vi "Project.Items.Add.vi"(8 "error in (no error)":errorcluster, 9 "Array":T1(array[cluster]), 10 "FPGA Target Name":string="FPGA Target", 11 "Path":path=path "C:/Users/Administrator/Desktop/Test Adding Memory to Project.lvproj") -> (0 "error out":errorcluster)   [LabVIEW 2015]
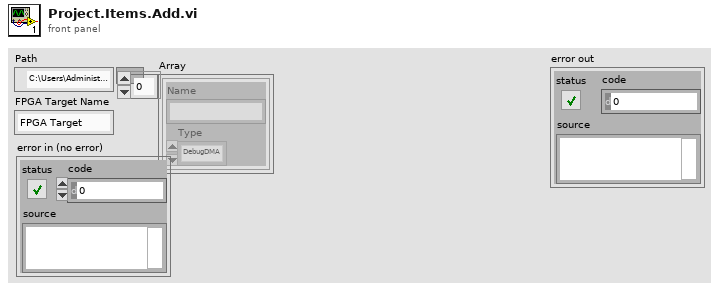
[diagram p1: front panel]
types:
  T1 = cluster{"Name":string, "Type":enum16{"DebugDMA", "Directional Memory", "Analog Replay Memory", "Pattern Generation Memory"}}[]
  T2 = enum16{"DebugDMA", "Directional Memory", "Analog Replay Memory", "Pattern Generation Memory"}
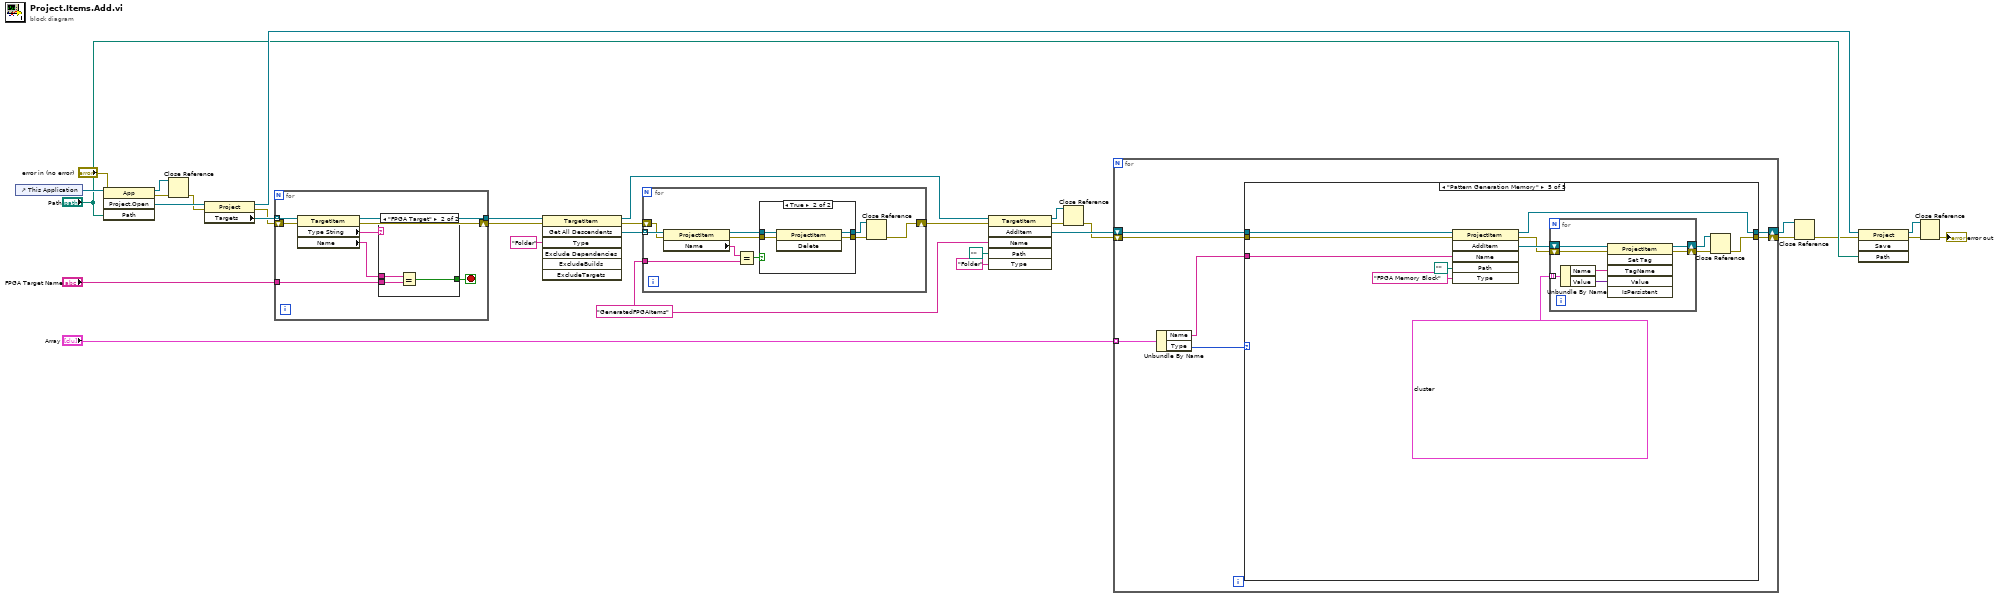
[diagram p0: block diagram]
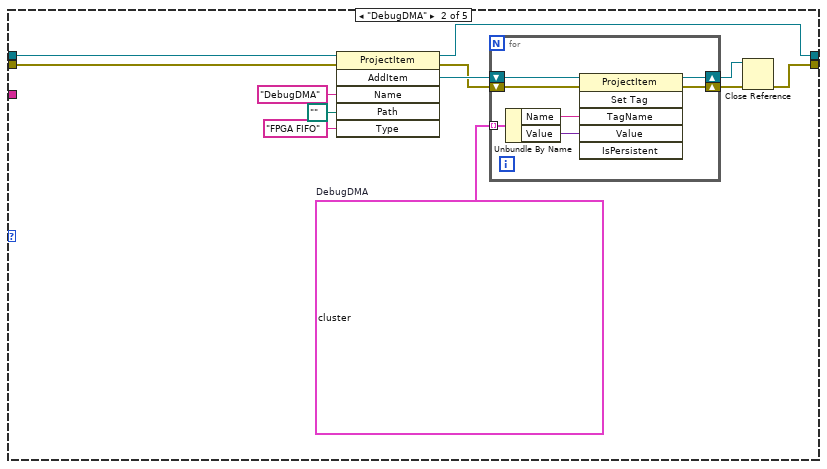
[diagram p3: hidden frame]
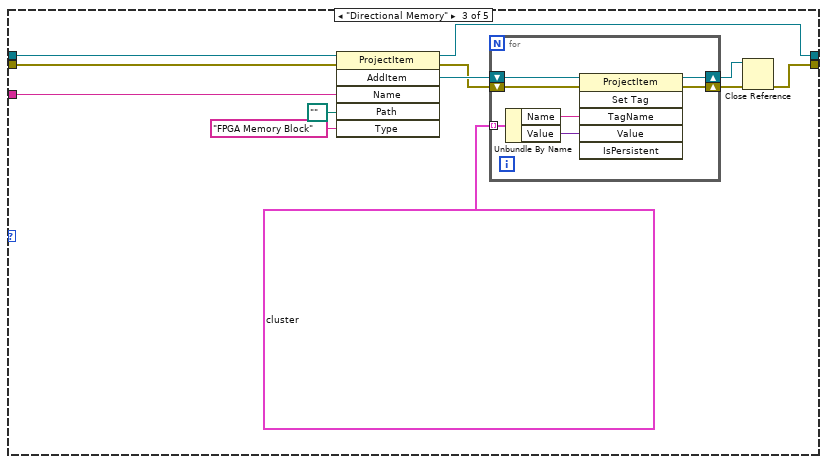
[diagram p4: hidden frame]
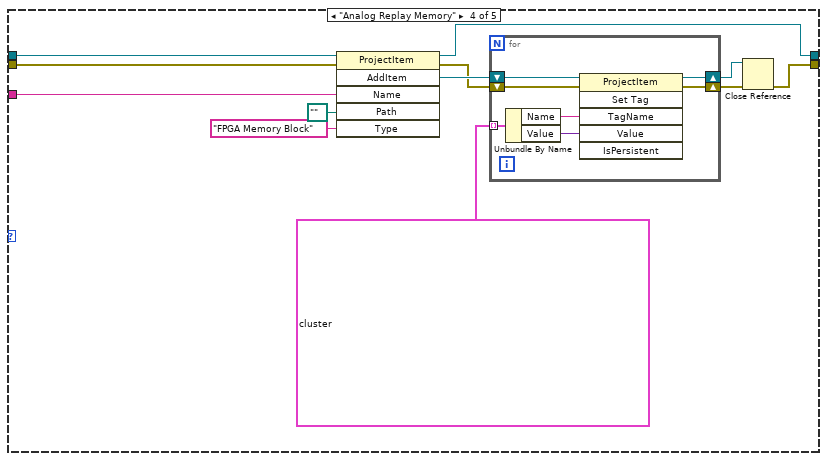
[diagram p5: hidden frame]
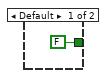
[diagram p6: hidden frame]
diagram:
  w12 = "GeneratedFPGAItems" ("Name")
  n1 = control-ref of="This Application"() -> (w32:refnum<vi>)
  n2 = invoke class="App" method="Project.Open"(reference=w32, error in="error in (no error)", "Path"="Path") -> (reference out=w19:refnum<vi>, error out=w21:errorcluster, "Project:Open"=w31:refnum<vi>)  [unwired: 1 in, 1 out]
  n3 = Close Reference(reference=w19, error in (no error)=w21) -> (error out=w20:errorcluster)
  n4 = property class="Project"(reference=w31, error in=w20) -> (reference out=w26:refnum<vi>, error out=w17:errorcluster, "Targets"=w18:refnum<vi>[])
  n5 = for {
    tunnel: w18 -> [w40] mode=indexing
    tunnel: "FPGA Target Name" -> [w39]
    shift-right: [w36] -> w16
    shift-left: w17 -> [w37]
    tunnel: [w35] -> w15
    stop <- w34 stop-if-true
    n6 = property class="TargetItem"(reference=w40, error in=w37) -> (reference out=w35:refnum<vi>, error out=w36:errorcluster, "Type String"=w33:string, "Name"=w38:string)
    n7 = case shown="\"FPGA Target\"" w33 {
      tunnel: w39 -> [_ w44]
      tunnel: w38 -> [_ w43]
      tunnel: [FALSE w42] -> w34
      frame Default {
      }
      frame "FPGA Target" {
        n8 = Equal?(x=w43, y=w44) -> (x = y?=w42:bool)
      }
    }
  }
  n9 = invoke class="TargetItem" method="Get All Descendents"(reference=w15, error in=w16, "Type"="Folder") -> (reference out=w13:refnum<vi>, error out=w22:errorcluster, "All Descendents"=w23:refnum<vi>[])  [unwired: 4 in, 4 out]
  n10 = for {
    tunnel: w23 -> [w54] mode=indexing
    shift-right: [w45] -> w28
    shift-left: w22 -> [w53]
    tunnel: w12 -> [w51]
    n11 = property class="ProjectItem"(reference=w54, error in=w53) -> (reference out=w50:refnum<vi>, error out=w49:errorcluster, "Name"=w52:string)
    n12 = Equal?(x=w52, y=w51) -> (x = y?=w48:bool)
    n13 = case shown="True" w48 {
      tunnel: w50 -> [w55 w60]
      tunnel: w49 -> [w56 w59]
      tunnel: [w56 w58] -> w46
      tunnel: [w55 w57] -> w47
      frame False {
      }
      frame True {
        n14 = invoke class="ProjectItem" method="Delete"(reference=w60, error in=w59) -> (reference out=w57:refnum<vi>, error out=w58:errorcluster)  [unwired: 1 in, 1 out]
      }
    }
    n15 = Close Reference(reference=w47, error in (no error)=w46) -> (error out=w45:errorcluster)
  }
  n16 = invoke class="TargetItem" method="AddItem"(reference=w13, error in=w28, "Name"=w12, "Path"=path "", "Type"="Folder") -> (reference out=w11:refnum<vi>, error out=w10:errorcluster, "AddItem"=w29:refnum<vi>)  [unwired: 1 in, 3 out]
  n17 = Close Reference(reference=w11, error in (no error)=w10) -> (error out=w9:errorcluster)
  n18 = for {
    shift-right: [w66] -> w5
    shift-left: w9 -> [w65]
    shift-right: [w64] -> w3
    shift-left: w29 -> [w67]
    tunnel: "Array" -> [w63] mode=indexing
    n19 = Unbundle By Name(w63) -> ("Name"=w61:string, "Type"=w62:T2)
    n20 = case shown="\"Pattern Generation Memory\"" w62 {
      tunnel: w67 -> [w68 w81 w100 w119 w138]
      tunnel: [w69 w70 w92 w111 w130] -> w66
      tunnel: w65 -> [w69 w75 w90 w108 w128]
      tunnel: [w68 w73 w95 w114 w133] -> w64
      tunnel: w61 -> [_ _ w89 w109 w127]
      frame Default {
      }
      frame "DebugDMA" {
        w77 = cluster{"Name":string, "Value":variant}[] [{"Name"="Actual Number of Elements", "Value"=variant(u32 1023)}, {"Name"="Arbitration for Read", "Value"=variant(u32 1)}, {"Name"="Arbitration for Write", "Value"=variant(u32 1)}, {"Name"="Control Logic", "Value"=variant(u32 0)}, {"Name"="Data Type", "Value"=variant(u32 11)}, {"Name"="Disable on Overflow/Underflow", "Value"=variant(bool FALSE)}, {"Name"="fifo.configuration", "Value"=variant(string "\"ControlLogic=0;NumberOfElements=1023;Type=2;ReadArbs=Arbitrate if Multiple Requestors Only;ElementsPerRead=1;WriteArbs=Arbitrate if Multiple Requestors Only;ElementsPerWrite=1;Implementation=2;FIFO;DataType=100080000000000100094009000353474C000100000000000000000000;DisableOnOverflowUnderflow=FALSE\"")}, {"Name"="fifo.configured", "Value"=variant(bool TRUE)}, {"Name"="fifo.projectItemValid", "Value"=variant(bool TRUE)}, {"Name"="fifo.valid", "Value"=variant(bool TRUE)}, {"Name"="fifo.version", "Value"=variant(i32 12)}, {"Name"="FPGA.PersistentID", "Value"=variant(string "{43D2C6D9-9E30-4F2C-9E9A-27A6F06ED45E}")}, {"Name"="Local", "Value"=variant(bool FALSE)}, {"Name"="Memory Type", "Value"=variant(u32 2)}, {"Name"="Number Of Elements Per Read", "Value"=variant(u32 1)}, {"Name"="Number Of Elements Per Write", "Value"=variant(u32 1)}, {"Name"="Requested Number of Elements", "Value"=variant(u32 1023)}, {"Name"="Type", "Value"=variant(u32 2)}, {"Name"="Type Descriptor", "Value"=variant(string "100080000000000100094009000353474C000100000000000000000000")}]  # DebugDMA
        n21 = invoke class="ProjectItem" method="AddItem"(reference=w81, error in=w75, "Name"="DebugDMA", "Path"=path "", "Type"="FPGA FIFO") -> (reference out=w73:refnum<vi>, error out=w74:errorcluster, "AddItem"=w78:refnum<vi>)  [unwired: 1 in, 3 out]
        n22 = for {
          shift-right: [w83] -> w71
          shift-left: w74 -> [w87]
          tunnel: w77 -> [w86] mode=indexing
          shift-right: [w82] -> w72
          shift-left: w78 -> [w88]
          n23 = Unbundle By Name(w86) -> ("Name"=w85:string, "Value"=w84:variant)
          n24 = invoke class="ProjectItem" method="Set Tag"(reference=w88, error in=w87, "TagName"=w85, "Value"=w84) -> (reference out=w82:refnum<vi>, error out=w83:errorcluster)  [unwired: 2 in, 4 out]
        }
        n25 = Close Reference(reference=w72, error in (no error)=w71) -> (error out=w70:errorcluster)
      }
      frame "Directional Memory" {
        n26 = invoke class="ProjectItem" method="AddItem"(reference=w100, error in=w90, "Name"=w89, "Path"=path "", "Type"="FPGA Memory Block") -> (reference out=w95:refnum<vi>, error out=w96:errorcluster, "AddItem"=w98:refnum<vi>)  [unwired: 1 in, 3 out]
        n27 = for {
          shift-right: [w102] -> w93
          shift-left: w96 -> [w106]
          tunnel: cluster{"Name":string, "Value":variant}[] [{"Name"="FPGA.PersistentID", "Value"=variant(string "{CD7EB185-1A87-4E78-8C08-5D9A1491F439}")}, {"Name"="fullEmulation", "Value"=variant(bool TRUE)}, {"Name"="Memory Latency", "Value"=variant(u32 1)}, {"Name"="Multiple Clock Domains", "Value"=variant(bool FALSE)}, {"Name"="NI.LV.FPGA.CompileConfigString", "Value"=variant(string "Actual Number of Elements=1024;ReadArbs=2;WriteArbs=2;Implementation=2;DataType=100080000000000100094006000355313600010000000000000000;InitDataHash=;DRAM Selection=DramBank0;DRAM Max Outstanding Requests=64;DRAM Include Byte Enables=FALSE;DRAM Grant Time=50;Interface Configuration=Read A-Write B;Multiple Clock Domains=FALSE;Memory Latency=1")}, {"Name"="NI.LV.FPGA.MEMORY.ActualNumberOfElements", "Value"=variant(u32 1024)}, {"Name"="NI.LV.FPGA.MEMORY.DataWidth", "Value"=variant(u32 6)}, {"Name"="NI.LV.FPGA.MEMORY.DramIncludeByteEnables", "Value"=variant(bool FALSE)}, {"Name"="NI.LV.FPGA.MEMORY.DramMaxOutstandingRequests", "Value"=variant(i32 64)}, {"Name"="NI.LV.FPGA.MEMORY.DramSelection", "Value"=variant(string "DramBank0")}, {"Name"="NI.LV.FPGA.MEMORY.Init", "Value"=variant(bool FALSE)}, {"Name"="NI.LV.FPGA.MEMORY.InitData", "Value"=variant(string "")}, {"Name"="NI.LV.FPGA.MEMORY.InitVIPath", "Value"=variant(string "")}, {"Name"="NI.LV.FPGA.MEMORY.InterfaceAArbitration", "Value"=variant(u32 2)}, {"Name"="NI.LV.FPGA.MEMORY.InterfaceBArbitration", "Value"=variant(u32 2)}, {"Name"="NI.LV.FPGA.MEMORY.InterfaceConfig", "Value"=variant(u32 0)}, {"Name"="NI.LV.FPGA.MEMORY.RequestedNumberOfElements", "Value"=variant(u32 1024)}, {"Name"="NI.LV.FPGA.MEMORY.Type", "Value"=variant(u32 2)}, {"Name"="NI.LV.FPGA.ScriptConfigString", "Value"=variant(string "Actual Number of Elements=1024;ReadArbs=2;WriteArbs=2;Implementation=2;DataType=100080000000000100094006000355313600010000000000000000;InitDataHash=;DRAM Selection=DramBank0;DRAM Max Outstanding Requests=64;DRAM Include Byte Enables=FALSE;DRAM Grant Time=50;Interface Configuration=Read A-Write B;Multiple Clock Domains=FALSE;Memory Latency=1Persist Memory ValuesTRUE;")}, {"Name"="NI.LV.FPGA.Valid", "Value"=variant(bool TRUE)}, {"Name"="NI.LV.FPGA.Version", "Value"=variant(i32 10)}, {"Name"="Type Descriptor", "Value"=variant(string "100080000000000100094006000355313600010000000000000000")}] ("Array 2") -> [w105] mode=indexing
          shift-right: [w101] -> w94
          shift-left: w98 -> [w107]
          n28 = Unbundle By Name(w105) -> ("Name"=w104:string, "Value"=w103:variant)
          n29 = invoke class="ProjectItem" method="Set Tag"(reference=w107, error in=w106, "TagName"=w104, "Value"=w103) -> (reference out=w101:refnum<vi>, error out=w102:errorcluster)  [unwired: 2 in, 4 out]
        }
        n30 = Close Reference(reference=w94, error in (no error)=w93) -> (error out=w92:errorcluster)
      }
      frame "Analog Replay Memory" {
        n31 = invoke class="ProjectItem" method="AddItem"(reference=w119, error in=w108, "Name"=w109, "Path"=path "", "Type"="FPGA Memory Block") -> (reference out=w114:refnum<vi>, error out=w115:errorcluster, "AddItem"=w117:refnum<vi>)  [unwired: 1 in, 3 out]
        n32 = for {
          shift-right: [w121] -> w112
          shift-left: w115 -> [w125]
          tunnel: cluster{"Name":string, "Value":variant}[] [{"Name"="FPGA.PersistentID", "Value"=variant(string "{CD7EB185-1A87-4E78-8C08-5D9A1491F439}")}, {"Name"="fullEmulation", "Value"=variant(bool TRUE)}, {"Name"="Memory Latency", "Value"=variant(u32 1)}, {"Name"="Multiple Clock Domains", "Value"=variant(bool FALSE)}, {"Name"="NI.LV.FPGA.CompileConfigString", "Value"=variant(string "Actual Number of Elements=16384;ReadArbs=2;WriteArbs=2;Implementation=2;DataType=100080000000000100094002000349313600010000000000000000;InitDataHash=;DRAM Selection=DramBank0;DRAM Max Outstanding Requests=64;DRAM Include Byte Enables=FALSE;DRAM Grant Time=50;Interface Configuration=Read A-Write B;Multiple Clock Domains=FALSE;Memory Latency=1")}, {"Name"="NI.LV.FPGA.MEMORY.ActualNumberOfElements", "Value"=variant(u32 16384)}, {"Name"="NI.LV.FPGA.MEMORY.DataWidth", "Value"=variant(u32 2)}, {"Name"="NI.LV.FPGA.MEMORY.DramIncludeByteEnables", "Value"=variant(bool FALSE)}, {"Name"="NI.LV.FPGA.MEMORY.DramMaxOutstandingRequests", "Value"=variant(i32 64)}, {"Name"="NI.LV.FPGA.MEMORY.DramSelection", "Value"=variant(string "DramBank0")}, {"Name"="NI.LV.FPGA.MEMORY.Init", "Value"=variant(bool FALSE)}, {"Name"="NI.LV.FPGA.MEMORY.InitData", "Value"=variant(string "")}, {"Name"="NI.LV.FPGA.MEMORY.InitVIPath", "Value"=variant(string "")}, {"Name"="NI.LV.FPGA.MEMORY.InterfaceAArbitration", "Value"=variant(u32 2)}, {"Name"="NI.LV.FPGA.MEMORY.InterfaceBArbitration", "Value"=variant(u32 2)}, {"Name"="NI.LV.FPGA.MEMORY.InterfaceConfig", "Value"=variant(u32 0)}, {"Name"="NI.LV.FPGA.MEMORY.RequestedNumberOfElements", "Value"=variant(u32 16384)}, {"Name"="NI.LV.FPGA.MEMORY.Type", "Value"=variant(u32 2)}, {"Name"="NI.LV.FPGA.ScriptConfigString", "Value"=variant(string "Actual Number of Elements=16384;ReadArbs=2;WriteArbs=2;Implementation=2;DataType=100080000000000100094002000349313600010000000000000000;InitDataHash=;DRAM Selection=DramBank0;DRAM Max Outstanding Requests=64;DRAM Include Byte Enables=FALSE;DRAM Grant Time=50;Interface Configuration=Read A-Write B;Multiple Clock Domains=FALSE;Memory Latency=1Persist Memory ValuesTRUE;")}, {"Name"="NI.LV.FPGA.Valid", "Value"=variant(bool TRUE)}, {"Name"="NI.LV.FPGA.Version", "Value"=variant(i32 10)}, {"Name"="Type Descriptor", "Value"=variant(string "100080000000000100094002000349313600010000000000000000")}] ("Array 2") -> [w124] mode=indexing
          shift-right: [w120] -> w113
          shift-left: w117 -> [w126]
          n33 = Unbundle By Name(w124) -> ("Name"=w123:string, "Value"=w122:variant)
          n34 = invoke class="ProjectItem" method="Set Tag"(reference=w126, error in=w125, "TagName"=w123, "Value"=w122) -> (reference out=w120:refnum<vi>, error out=w121:errorcluster)  [unwired: 2 in, 4 out]
        }
        n35 = Close Reference(reference=w113, error in (no error)=w112) -> (error out=w111:errorcluster)
      }
      frame "Pattern Generation Memory" {
        n36 = invoke class="ProjectItem" method="AddItem"(reference=w138, error in=w128, "Name"=w127, "Path"=path "", "Type"="FPGA Memory Block") -> (reference out=w133:refnum<vi>, error out=w134:errorcluster, "AddItem"=w136:refnum<vi>)  [unwired: 1 in, 3 out]
        n37 = for {
          shift-right: [w140] -> w131
          shift-left: w134 -> [w144]
          tunnel: cluster{"Name":string, "Value":variant}[] [{"Name"="FPGA.PersistentID", "Value"=variant(string "{CD7EB185-1A87-4E78-8C08-5D9A1491F439}")}, {"Name"="fullEmulation", "Value"=variant(bool TRUE)}, {"Name"="Memory Latency", "Value"=variant(u32 1)}, {"Name"="Multiple Clock Domains", "Value"=variant(bool FALSE)}, {"Name"="NI.LV.FPGA.CompileConfigString", "Value"=variant(string "Actual Number of Elements=1024;ReadArbs=2;WriteArbs=2;Implementation=2;DataType=100080000000000100094006000355313600010000000000000000;InitDataHash=;DRAM Selection=DramBank0;DRAM Max Outstanding Requests=64;DRAM Include Byte Enables=FALSE;DRAM Grant Time=50;Interface Configuration=Read A-Write B;Multiple Clock Domains=FALSE;Memory Latency=1")}, {"Name"="NI.LV.FPGA.MEMORY.ActualNumberOfElements", "Value"=variant(u32 1024)}, {"Name"="NI.LV.FPGA.MEMORY.DataWidth", "Value"=variant(u32 6)}, {"Name"="NI.LV.FPGA.MEMORY.DramIncludeByteEnables", "Value"=variant(bool FALSE)}, {"Name"="NI.LV.FPGA.MEMORY.DramMaxOutstandingRequests", "Value"=variant(i32 64)}, {"Name"="NI.LV.FPGA.MEMORY.DramSelection", "Value"=variant(string "DramBank0")}, {"Name"="NI.LV.FPGA.MEMORY.Init", "Value"=variant(bool FALSE)}, {"Name"="NI.LV.FPGA.MEMORY.InitData", "Value"=variant(string "")}, {"Name"="NI.LV.FPGA.MEMORY.InitVIPath", "Value"=variant(string "")}, {"Name"="NI.LV.FPGA.MEMORY.InterfaceAArbitration", "Value"=variant(u32 2)}, {"Name"="NI.LV.FPGA.MEMORY.InterfaceBArbitration", "Value"=variant(u32 2)}, {"Name"="NI.LV.FPGA.MEMORY.InterfaceConfig", "Value"=variant(u32 0)}, {"Name"="NI.LV.FPGA.MEMORY.RequestedNumberOfElements", "Value"=variant(u32 1024)}, {"Name"="NI.LV.FPGA.MEMORY.Type", "Value"=variant(u32 2)}, {"Name"="NI.LV.FPGA.ScriptConfigString", "Value"=variant(string "Actual Number of Elements=1024;ReadArbs=2;WriteArbs=2;Implementation=2;DataType=100080000000000100094006000355313600010000000000000000;InitDataHash=;DRAM Selection=DramBank0;DRAM Max Outstanding Requests=64;DRAM Include Byte Enables=FALSE;DRAM Grant Time=50;Interface Configuration=Read A-Write B;Multiple Clock Domains=FALSE;Memory Latency=1Persist Memory ValuesTRUE;")}, {"Name"="NI.LV.FPGA.Valid", "Value"=variant(bool TRUE)}, {"Name"="NI.LV.FPGA.Version", "Value"=variant(i32 10)}, {"Name"="Type Descriptor", "Value"=variant(string "100080000000000100094006000355313600010000000000000000")}] ("Array 2") -> [w143] mode=indexing
          shift-right: [w139] -> w132
          shift-left: w136 -> [w145]
          n38 = Unbundle By Name(w143) -> ("Name"=w142:string, "Value"=w141:variant)
          n39 = invoke class="ProjectItem" method="Set Tag"(reference=w145, error in=w144, "TagName"=w142, "Value"=w141) -> (reference out=w139:refnum<vi>, error out=w140:errorcluster)  [unwired: 2 in, 4 out]
        }
        n40 = Close Reference(reference=w132, error in (no error)=w131) -> (error out=w130:errorcluster)
      }
    }
  }
  n41 = Close Reference(reference=w3, error in (no error)=w5) -> (error out=w4:errorcluster)
  n42 = invoke class="Project" method="Save"(reference=w26, error in=w4, "Path"="Path") -> (reference out=w8:refnum<vi>, error out=w7:errorcluster)  [unwired: 1 in, 2 out]
  n43 = Close Reference(reference=w8, error in (no error)=w7) -> (error out=→"error out":errorcluster)
